vi "Check Abort or Pause Message During Execution Task.vi"(8 "error in (no error)":errorcluster, 11 "System Actor in":refnum<class "System Actor.lvclass">) -> (0 "error out":errorcluster, 2 "Abort?":bool, 3 "System Actor out":refnum<class "System Actor.lvclass">)   [LabVIEW 2019, in "System Actor.lvclass"]
uses:
  System Actor.lvclass
  Message/Message.lvclass/Message.ctl
  Message/Public Data/Read CMD Type.vi
  Message/Public Data/Read General CMD.vi
  Message/Message.lvclass
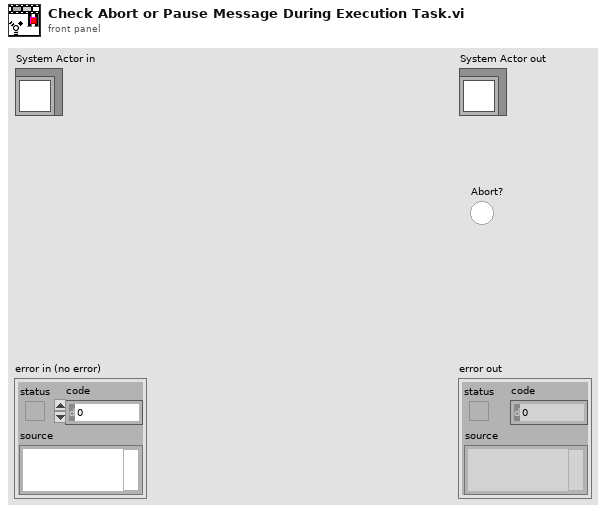
[diagram p1: front panel]
types:
  T1 = typedef "CMD Type.ctl" = enum16{"None", "General CMD", "1st CMD", "2nd CMD", "3rd CMD", "4th CMD", "5th CMD", "6th CMD", "7th CMD"}
  T2 = typedef "General CMD.ctl" = enum16{"None", "Stop", "Abort", "Running Task", "Running Batch Tasks", "Task Self Running", "Emergency Stop", "Subscribe", "UnSubscribe", "Pause"}
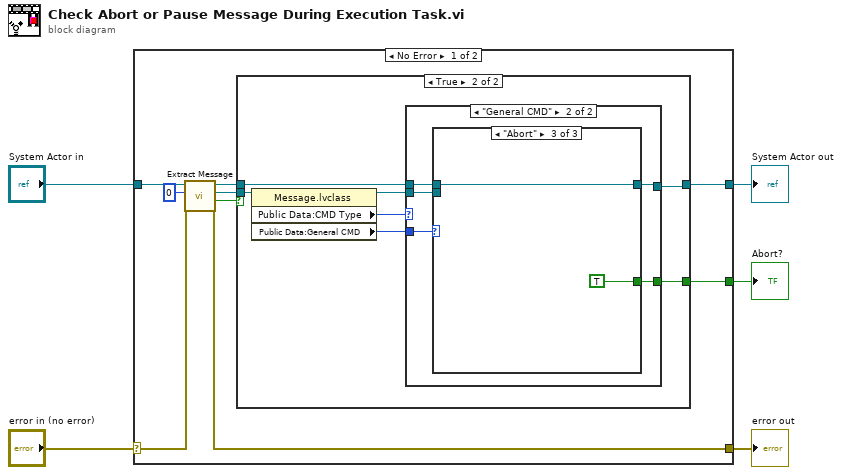
[diagram p0: block diagram]
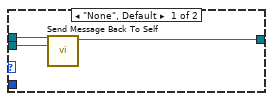
[diagram p3: hidden frame]
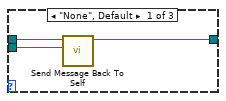
[diagram p4: hidden frame]
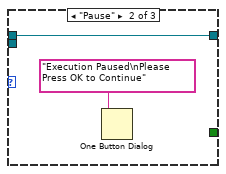
[diagram p5: hidden frame]
diagram:
  n1 = case shown="No Error" "error in (no error)" {
    selector: "error in (no error)" -> [w12 w39]
    tunnel: [w11 w39] -> w4
    tunnel: [w8 w38] -> w2
    tunnel: "System Actor in" -> [w14 w38]
    tunnel: [w6 _] -> w1
    frame No Error {
      n2 = call-dynamic "Extract Message.vi"("error in (no error)"=w12, "Wait"=0, "System Actor in"=w14) -> ("error out"=w11:errorcluster, "Valid"=w10:bool, "Message Out"=w7:refnum<class "Message.lvclass">, "System Actor out"=w9:refnum<class "System Actor.lvclass">)  [unwired: 5 in]
      n3 = case shown="True" w10 {
        tunnel: w9 -> [w15 w19]
        tunnel: [w15 w18] -> w8
        tunnel: w7 -> [_ w22]
        tunnel: [_ w16] -> w6
        frame False {
        }
        frame True {
          n4 = property class="Message.lvclass"(reference=w22) -> (reference out=w20:refnum<class "Message.lvclass">, "Public Data:CMD Type"=w21:T1, "Public Data:General CMD"=w17:T2)  [unwired: 1 in, 1 out]
          n5 = case shown="\"General CMD\"" w21 {
            tunnel: w20 -> [w24 w27]
            tunnel: w19 -> [w25 w29]
            tunnel: [w23 w28] -> w18
            tunnel: w17 -> [_ w30]
            tunnel: [_ w26] -> w16
            frame "None", Default {
              n6 = call "Send Message Back To Self.vi"("Message In"=w24, "System Actor in"=w25) -> ("System Actor out"=w23:refnum<class "System Actor.lvclass">)  [unwired: 8 in, 1 out]
            }
            frame "General CMD" {
              n7 = case shown="\"Abort\"" w30 {
                tunnel: w29 -> [w33 w35 w37]
                tunnel: [w32 w35 w37] -> w28
                tunnel: w27 -> [w31 _ _]
                tunnel: [_ _ TRUE ("Abort?")] -> w26
                frame "None", Default {
                  n8 = call "Send Message Back To Self.vi"("Message In"=w31, "System Actor in"=w33) -> ("System Actor out"=w32:refnum<class "System Actor.lvclass">)  [unwired: 8 in, 1 out]
                }
                frame "Pause" {
                  n9 = One Button Dialog(message="Execution Paused\nPlease Press OK to Continue") -> ()  [unwired: 1 in, 1 out]
                }
                frame "Abort" {
                }
              }
            }
          }
        }
      }
    }
    frame Error {
    }
  }
  "error out" <- w4
  "System Actor out" <- w2
  "Abort?" <- w1
